vi "Remove Question Mark.vi"(1 "Label In":string) -> (0 "Label (\"?\" removed from end)":string)   [LabVIEW 2011, in "Messenging.lvlib" / "MSG.lvclass"]
uses:
  MSG.lvclass
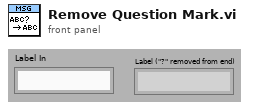
[diagram p1: front panel]
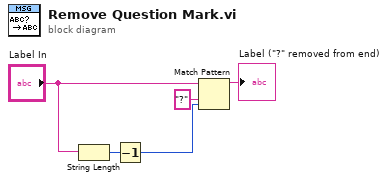
[diagram p0: block diagram]
diagram:
  n1 = String Length(string="Label In") -> (length=w4:i32)
  n2 = Decrement(x=w4) -> (x-1=w3:i32)
  n3 = Match Pattern(string="Label In", regular expression="?", offset (0)=w3) -> (before substring=→"Label (\"?\" removed from end)":string)  [unwired: 3 out]
